vi "Model - Set Invalid Login.vi"(8 "error in (no error)":errorcluster, 10 "Invalid login":i16, 11 "View Model":T1) -> (0 "error out":errorcluster, 3 "View Model":T1)   [LabVIEW 2017]
doc: "Get current and next ATM controller states values from DVR."
uses:
  Controls/View Model.ctl
  Error Handler/Controls/Error Model.ctl
  Error Handler/Controls/Error Data.ctl
  Error Handler/Controls/Error Type.ctl
  Controls/Shared Model.ctl
  Configuration/Controls/Config Model.ctl
  Configuration/Controls/Config CMD.ctl
  Configuration/Controls/Config Data.ctl
  ATM Controller/Controls/Controller Model.ctl
  ATM Controller/Controls/Controller Overhead.ctl
  ATM Controller/Controls/Controller States.ctl
  ATM Controller/Controls/Controller Message Data.ctl
  ATM Controller/Controls/Controller Message Name.ctl
  ATM Controller/Controls/Controller CMD.ctl
  Views/User Console View/Controls/User Console - Transaction Enum.ctl
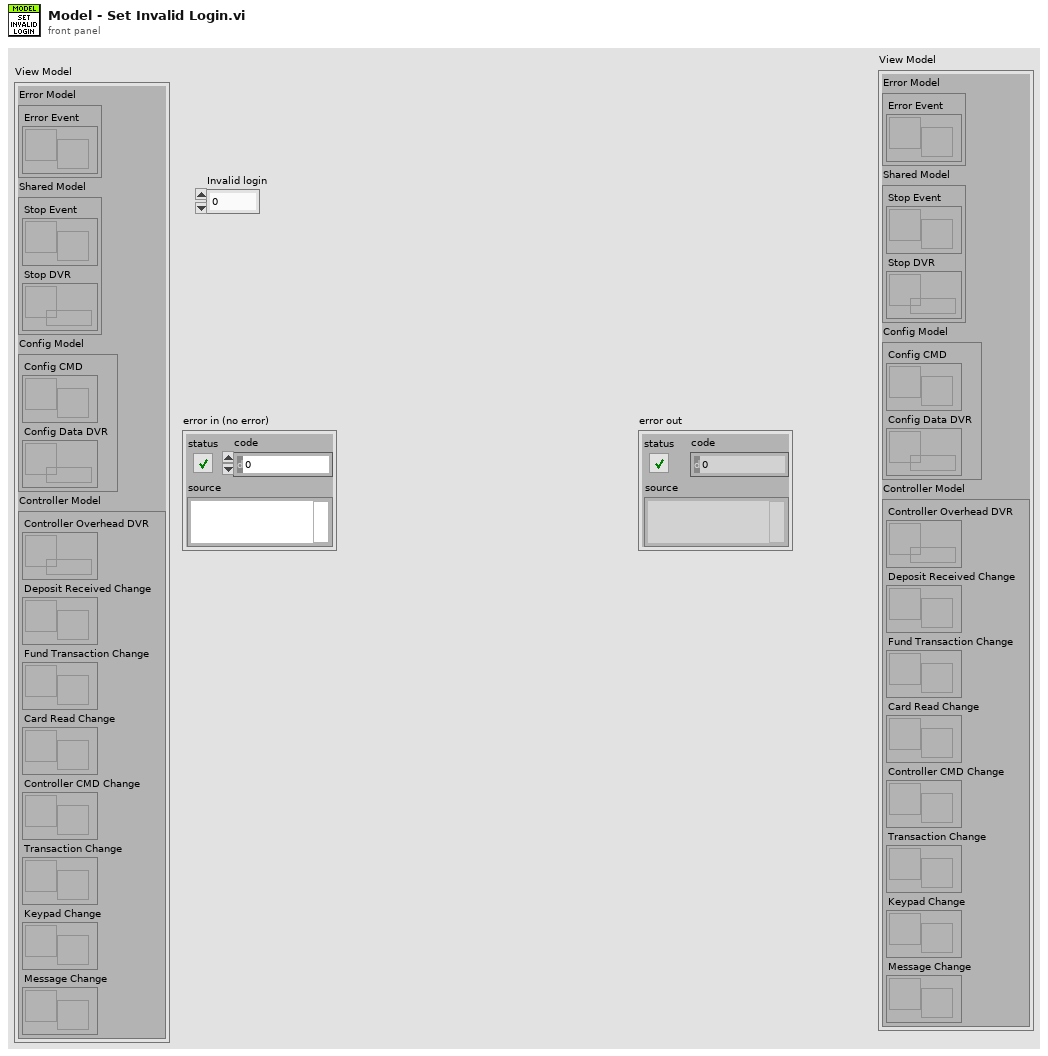
[diagram p1: front panel]
types:
  T1 = typedef "View Model.ctl" = cluster{"Error Model":T2, "Shared Model":T3, "Config Model":T4, "Controller Model":T5}
  T2 = typedef "Error Model.ctl" = cluster{"Error Event":refnum<user-event>}
  T3 = typedef "Shared Model.ctl" = cluster{"Stop Event":refnum<user-event>, "Stop DVR":refnum<data-value>}
  T4 = typedef "Config Model.ctl" = cluster{"Config CMD":refnum<user-event>, "Config Data DVR":refnum<data-value>}
  T5 = typedef "Controller Model.ctl" = cluster{"Controller Overhead DVR":refnum<data-value>, "Deposit Received Change":refnum<user-event>, "Fund Transaction Change":refnum<user-event>, "Card Read Change":refnum<user-event>, "Controller CMD Change":refnum<user-event>, "Transaction Change":refnum<user-event>, "Keypad Change":refnum<user-event>, "Message Change":refnum<user-event>}
  T6 = typedef "Controller Overhead.ctl" = cluster{"Account found":bool, "Current State":T7, "Next State":T7, "Inactivity Time":dbl, "Account Number":dbl, "Deposit Amount":dbl, "Withdrawal Amount":dbl, "Message Data List":T8[], "Invalid login":i16}
  T7 = typedef "Controller States.ctl" = enum16{"Idle", "Init", "Display Message", "Login", "Balance Inquiry", "Deposit", "Withdrawal", "Fast Cash", "Terminate"}
  T8 = typedef "Controller Message Data.ctl" = cluster{"Transaction":string, "Message":string, "Card Read":bool, "Message Name":T9}
  T9 = typedef "Controller Message Name.ctl" = enum16{"Welcome", "Login", "Idle", "Invalid Login", "Terminate", "Deposit", "Withdrawal", "Fast Cash", "Withdrawal Complete", "Withdrawal Failed", "Balance Inquiry"}
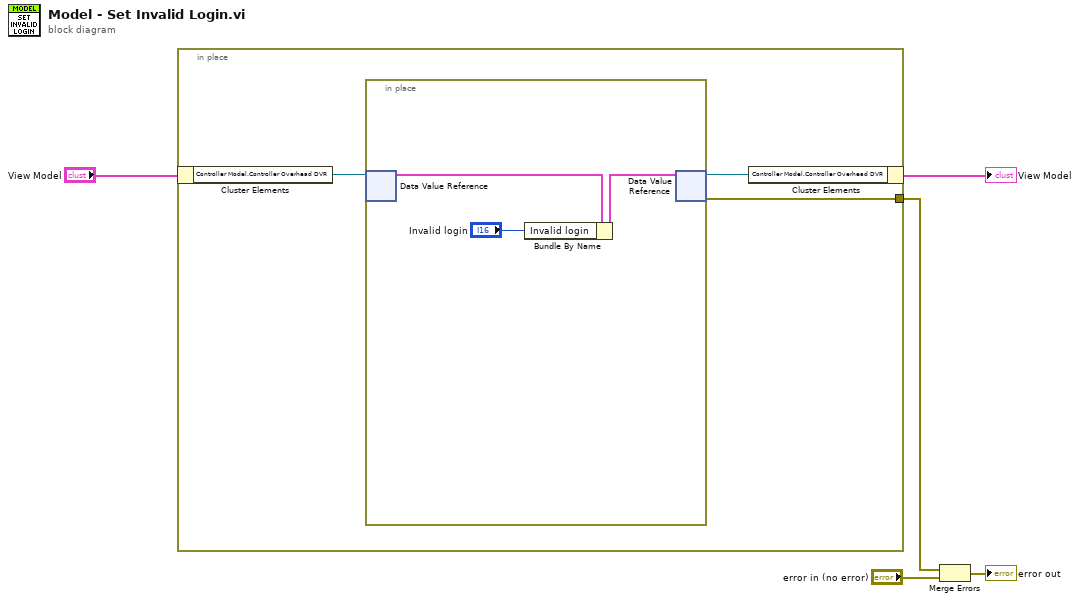
[diagram p0: block diagram]
diagram:
  n1 = in-place {
    in-place-border: [w6] -> w2
    n2 = in-place-cluster #1("View Model") -> ("Controller Model.Controller Overhead DVR"=w8:refnum<data-value>)
    n3 = in-place {
      n4 = in-place-dvr #2(w8) -> (w11:T6)  [unwired: 1 out]
      n5 = Bundle By Name(cluster=w11, "Invalid login"="Invalid login") -> (w10:T6)
      n6 = in-place-dvr #2(w10) -> (w7:refnum<data-value>, w6:errorcluster)
    }
    n7 = in-place-cluster #1("Controller Model.Controller Overhead DVR"=w7) -> (→"View Model":T1)
  }
  n8 = Merge Errors(w2, "error in (no error)") -> (→"error out":errorcluster)
